vi "Append Table Row Contents to Word.vi"(0 "report in":refnum<class "NI_report.lvclass">, 5 "table row contents":string[](array[string]), 9 "table index (-1)":i16=-1, 11 "error in (no error)":errorcluster, 12 "row#":i32) -> (4 "report out":refnum<class "NI_report.lvclass">, 15 "error out":errorcluster)   [LabVIEW 2018, in "WordReportGeneration.lvlib" / "Word_Report.lvclass"]
uses:
  Word_Report.lvclass
  <vilib>/Utility/NIReport.llb/NI_report.lvclass
  <vilib>/addons/_office/word.llb/Word Edit Cell ([str]).vi
  <vilib>/Utility/NIReport.llb/Word/NI_Word.lvclass
  <vilib>/addons/_office/NI_ReportGenerationToolkit.lvlib
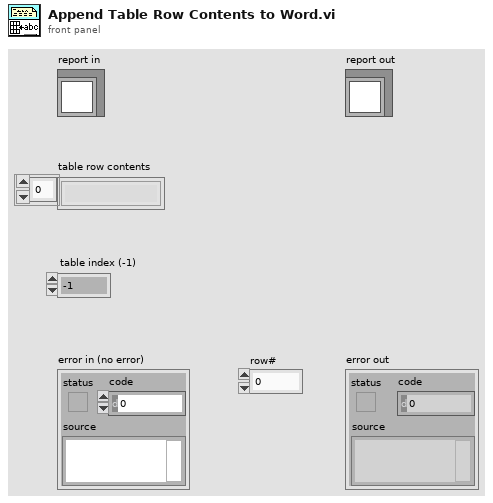
[diagram p1: front panel]
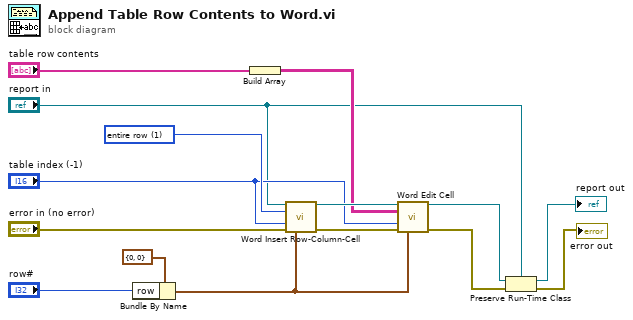
[diagram p0: block diagram]
diagram:
  w15 = u16 1 items=["shift cells right", "entire row", "entire column"] ("mode (entire column)")
  n1 = Bundle By Name(cluster=cluster{"row":i32, "column":i32} {"row"=0, "column"=0} ("start (0, 0)"), "row"="row#") -> (w7:cluster{"row":i32, "column":i32})
  n2 = Build Array("table row contents") -> (w9:string[][])
  n3 = call <vilib>:"Word Insert Row-Column-Cell.vi"("report in"="report in", "mode (entire column)"=w15, "table index (-1)"="table index (-1)", "error in (no error)"="error in (no error)", "start (0, 0)"=w7) -> ("report out"=w13:refnum<class "NI_report.lvclass">, "error out"=w12:errorcluster)  [unwired: 9 in]
  n4 = call-poly <vilib>:"Word Edit Cell.vi"("report in"=w13, "value"=w9, "table index (-1)"="table index (-1)", "error in (no error)"=w12, "start (0, 0)"=w7) -> ("report out"=w4:refnum<class "NI_report.lvclass">, "error out"=w2:errorcluster)  [unwired: 9 in]
  n5 = Preserve Run-Time Class(object in=w4, error in=w2, 2:"report in") -> (object out=→"report out":refnum<class "NI_report.lvclass">, error out=→"error out":errorcluster)
